vi "CRYImp wiz decide action new.vi"(7 "Iteration":i32, 10 "New controls":T1, 11 "Old controls":T1) -> (3 "Frames to run":string[](array[string]))   [LabVIEW 2013]
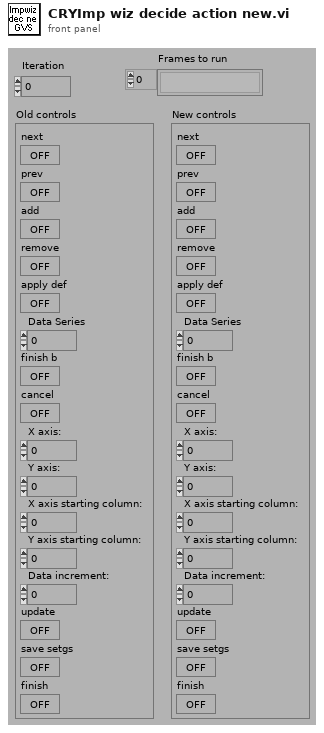
[diagram p1: front panel]
types:
  T1 = cluster{"next":bool, "prev":bool, "add":bool, "remove":bool, "apply def":bool, "Data Series":i32, "finish b":bool, "cancel":bool, "X axis:":i32, "Y axis:":i32, "X axis starting column:":i32, "Y axis starting column:":i32, "Data increment:":i32, "update":bool, "save setgs":bool, "finish":bool}
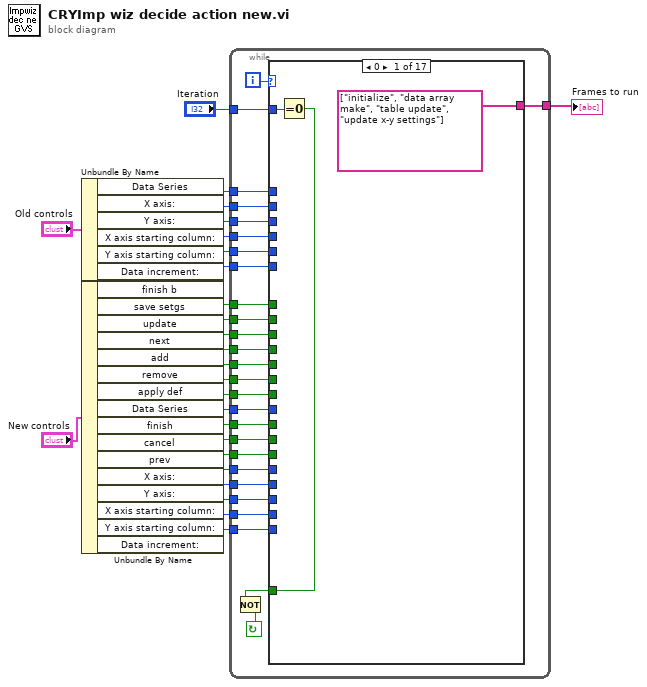
[diagram p0: block diagram]
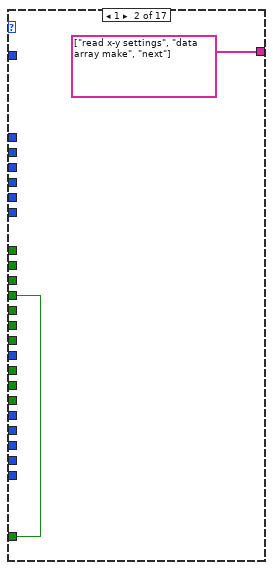
[diagram p2: hidden frame]
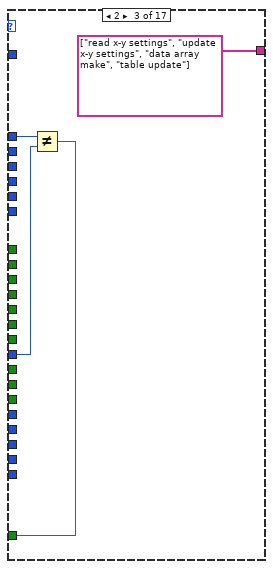
[diagram p3: hidden frame]
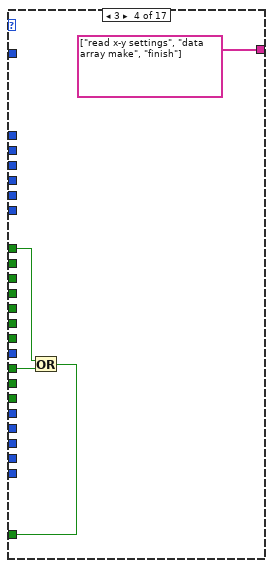
[diagram p4: hidden frame]
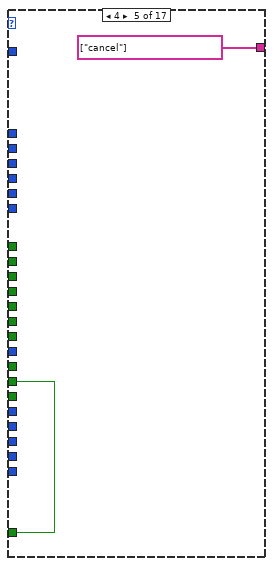
[diagram p5: hidden frame]
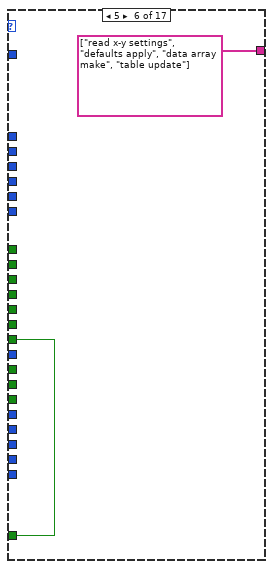
[diagram p6: hidden frame]
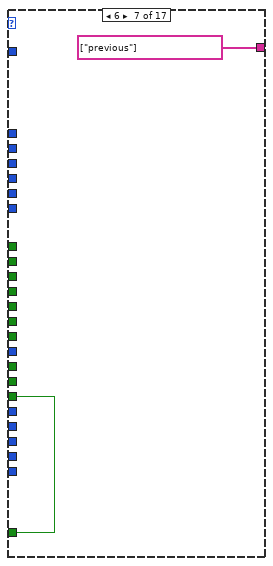
[diagram p7: hidden frame]
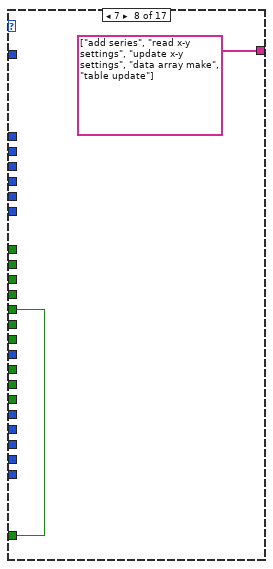
[diagram p8: hidden frame]
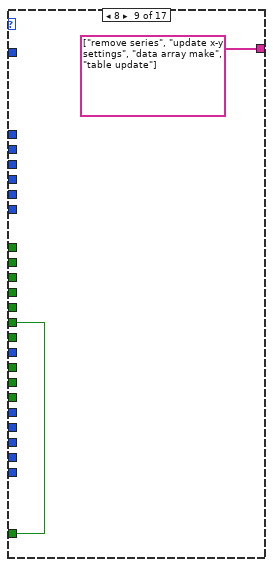
[diagram p9: hidden frame]
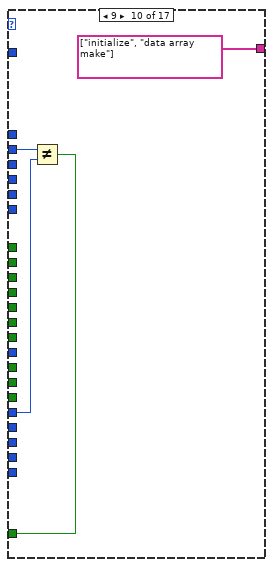
[diagram p10: hidden frame]
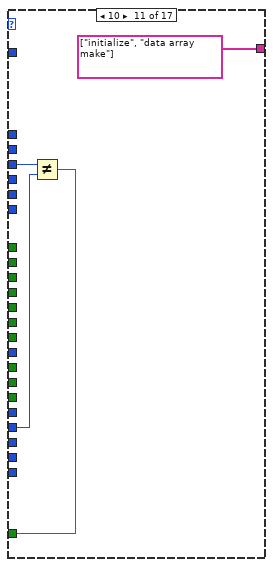
[diagram p11: hidden frame]
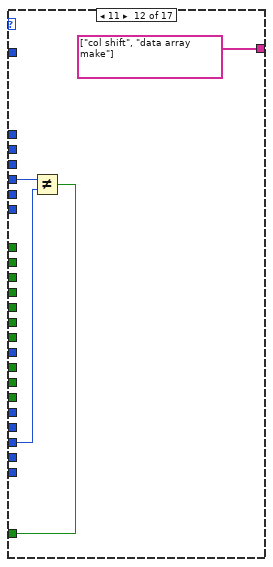
[diagram p12: hidden frame]
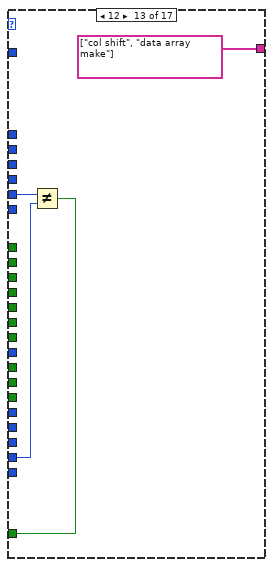
[diagram p13: hidden frame]
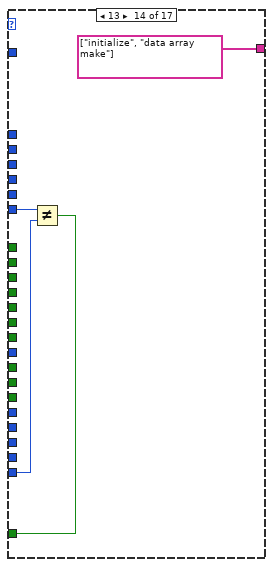
[diagram p14: hidden frame]
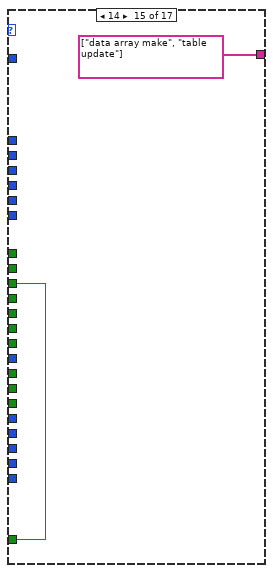
[diagram p15: hidden frame]
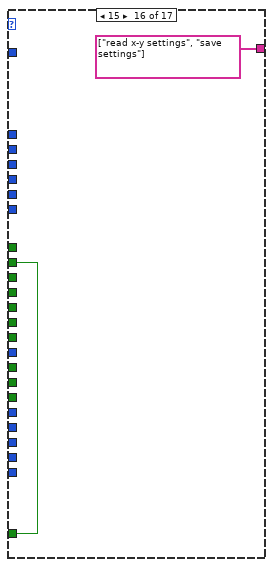
[diagram p16: hidden frame]
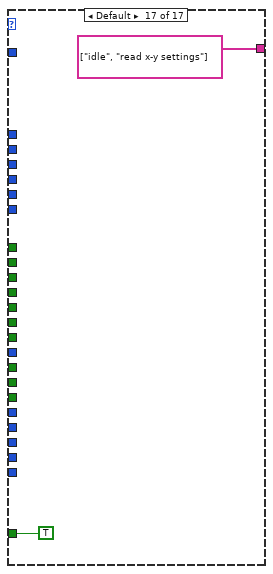
[diagram p17: hidden frame]
diagram:
  n1 = Unbundle By Name("Old controls") -> ("Data Series"=w23:i32, "X axis:"=w13:i32, "Y axis:"=w11:i32, "X axis starting column:"=w9:i32, "Y axis starting column:"=w8:i32, "Data increment:"=w7:i32)
  n2 = Unbundle By Name("New controls") -> ("finish b"=w1:bool, "save setgs"=w2:bool, "update"=w3:bool, "next"=w22:bool, "add"=w21:bool, "remove"=w20:bool, "apply def"=w19:bool, "Data Series"=w18:i32, "finish"=w17:bool, "cancel"=w16:bool, "prev"=w14:bool, "X axis:"=w12:i32, "Y axis:"=w10:i32, "X axis starting column:"=w6:i32, "Y axis starting column:"=w5:i32, "Data increment:"=w4:i32)
  n3 = while {
    tunnel: w1 -> [w27]
    tunnel: w2 -> [w28]
    tunnel: w3 -> [w29]
    tunnel: w4 -> [w30]
    tunnel: w5 -> [w31]
    tunnel: w6 -> [w32]
    tunnel: w7 -> [w33]
    tunnel: w8 -> [w34]
    tunnel: w9 -> [w35]
    tunnel: w10 -> [w36]
    tunnel: w11 -> [w37]
    tunnel: w12 -> [w38]
    tunnel: w13 -> [w39]
    tunnel: w14 -> [w40]
    tunnel: [w41] -> w15
    tunnel: w16 -> [w44]
    tunnel: w17 -> [w45]
    tunnel: w18 -> [w46]
    tunnel: w19 -> [w47]
    tunnel: w20 -> [w48]
    tunnel: w21 -> [w49]
    tunnel: w22 -> [w50]
    tunnel: w23 -> [w51]
    tunnel: "Iteration" -> [w52]
    i -> [w53]
    stop <- w42 continue-if-true
    n4 = case shown="0" w53 {
      tunnel: w52 -> [w56 _ _ _ _ _ _ _ _ _ _ _ _ _ _ _ _]
      tunnel: w51 -> [_ _ w61 _ _ _ _ _ _ _ _ _ _ _ _ _ _]
      tunnel: w50 -> [_ w58 _ _ _ _ _ _ _ _ _ _ _ _ _ _ _]
      tunnel: w49 -> [_ _ _ _ _ _ _ w74 _ _ _ _ _ _ _ _ _]
      tunnel: w48 -> [_ _ _ _ _ _ _ _ w76 _ _ _ _ _ _ _ _]
      tunnel: w47 -> [_ _ _ _ _ w69 _ _ _ _ _ _ _ _ _ _ _]
      tunnel: w46 -> [_ _ w60 _ _ _ _ _ _ _ _ _ _ _ _ _ _]
      tunnel: w45 -> [_ _ _ w65 _ _ _ _ _ _ _ _ _ _ _ _ _]
      tunnel: w44 -> [_ _ _ _ w67 _ _ _ _ _ _ _ _ _ _ _ _]
      tunnel: [w55 w58 w59 w63 w67 w69 w71 w74 w76 w79 w83 w87 w91 w95 w98 w100 TRUE] -> w43
      tunnel: [string[] ["initialize", "data array make", "table update", "update x-y settings"] string[] ["read x-y settings", "data array make", "next"] string[] ["read x-y settings", "update x-y settings", "data array make", "table update"] string[] ["read x-y settings", "data array make", "finish"] string[] ["cancel"] string[] ["read x-y settings", "defaults apply", "data array make", "table update"] string[] ["previous"] string[] ["add series", "read x-y settings", "update x-y settings", "data array make", "table update"] string[] ["remove series", "update x-y settings", "data array make", "table update"] string[] ["initialize", "data array make"] string[] ["initialize", "data array make"] string[] ["col shift", "data array make"] string[] ["col shift", "data array make"] string[] ["initialize", "data array make"] string[] ["data array make", "table update"] string[] ["read x-y settings", "save settings"] string[] ["idle", "read x-y settings"]] -> w41
      tunnel: w40 -> [_ _ _ _ _ _ w71 _ _ _ _ _ _ _ _ _ _]
      tunnel: w39 -> [_ _ _ _ _ _ _ _ _ w78 _ _ _ _ _ _ _]
      tunnel: w38 -> [_ _ _ _ _ _ _ _ _ w77 _ _ _ _ _ _ _]
      tunnel: w37 -> [_ _ _ _ _ _ _ _ _ _ w82 _ _ _ _ _ _]
      tunnel: w36 -> [_ _ _ _ _ _ _ _ _ _ w81 _ _ _ _ _ _]
      tunnel: w35 -> [_ _ _ _ _ _ _ _ _ _ _ w86 _ _ _ _ _]
      tunnel: w34 -> [_ _ _ _ _ _ _ _ _ _ _ _ w90 _ _ _ _]
      tunnel: w33 -> [_ _ _ _ _ _ _ _ _ _ _ _ _ w94 _ _ _]
      tunnel: w32 -> [_ _ _ _ _ _ _ _ _ _ _ w85 _ _ _ _ _]
      tunnel: w31 -> [_ _ _ _ _ _ _ _ _ _ _ _ w89 _ _ _ _]
      tunnel: w30 -> [_ _ _ _ _ _ _ _ _ _ _ _ _ w93 _ _ _]
      tunnel: w29 -> [_ _ _ _ _ _ _ _ _ _ _ _ _ _ w98 _ _]
      tunnel: w28 -> [_ _ _ _ _ _ _ _ _ _ _ _ _ _ _ w100 _]
      tunnel: w27 -> [_ _ _ w64 _ _ _ _ _ _ _ _ _ _ _ _ _]
      frame 0 {
        n5 = Equal To 0?(x=w56) -> (x = 0?=w55:bool)
      }
      frame 1 {
      }
      frame 2 {
        n6 = Not Equal?(x=w61, y=w60) -> (x != y?=w59:bool)
      }
      frame 3 {
        n7 = Or(x=w64, y=w65) -> (x .or. y?=w63:bool)
      }
      frame 4 {
      }
      frame 5 {
      }
      frame 6 {
      }
      frame 7 {
      }
      frame 8 {
      }
      frame 9 {
        n8 = Not Equal?(x=w78, y=w77) -> (x != y?=w79:bool)
      }
      frame 10 {
        n9 = Not Equal?(x=w82, y=w81) -> (x != y?=w83:bool)
      }
      frame 11 {
        n10 = Not Equal?(x=w86, y=w85) -> (x != y?=w87:bool)
      }
      frame 12 {
        n11 = Not Equal?(x=w90, y=w89) -> (x != y?=w91:bool)
      }
      frame 13 {
        n12 = Not Equal?(x=w94, y=w93) -> (x != y?=w95:bool)
      }
      frame 14 {
      }
      frame 15 {
      }
      frame Default {
      }
    }
    n13 = Not(x=w43) -> (.not. x?=w42:bool)
  }
  "Frames to run" <- w15
